vi "XLP80_Datalog_CreateFilename.vi"(8 "error in":errorcluster) -> (0 "error out":errorcluster caption="error in", 3 "Path":path, 5 "LogStartTime":dbl)   [LabVIEW 2021]
uses:
  XLP80_General_Libs/WL_Libs_V14.25/WL_Datalog_V14.00.llb/WL_Datalog_Global.vi
  XLP80_Globals/Globals_Settings_XLP80.vi
panel:
  out "x+1":i32
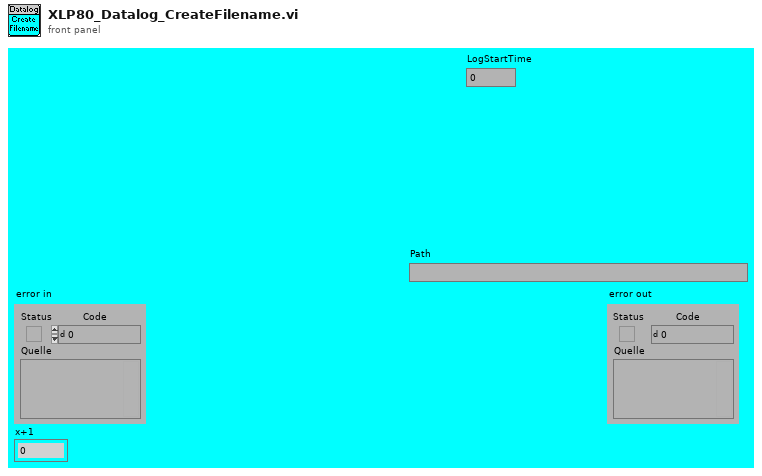
[diagram p1: front panel]
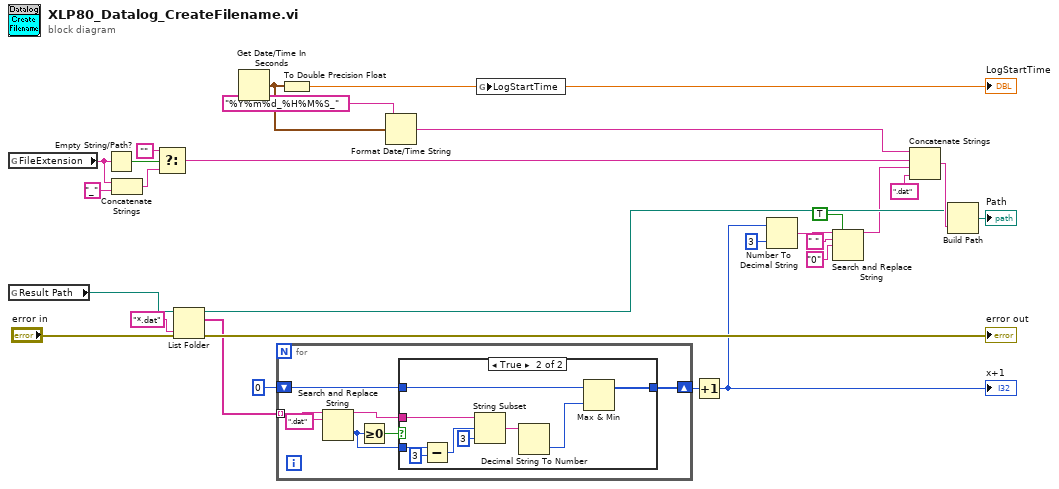
[diagram p0: block diagram]
diagram:
  n1 = global read "WL_Datalog_Global.vi" "FileExtension"() -> (w10:string)
  n2 = global read "Globals_Settings_XLP80.vi" "Result Path"() -> (w3:path)
  n3 = Empty String/Path?(string/path=w10) -> (empty?=w25:bool)
  n4 = Concatenate Strings(w10, "_" ("string")) -> (w24:string)
  n5 = Select(t="", s=w25, f=w24) -> (s? t:f=w1:string)
  n6 = List Folder(path=w3, pattern="*.dat", error in="error in") -> (path out=w13:path, filenames=w6:string[], error out=→"error out":errorcluster)  [unwired: 1 in, 1 out]
  n7 = Get Date/Time In Seconds() -> (seconds since 1Jan1904=w27:timestamp)
  n8 = for {
    tunnel: w6 -> [w35] mode=indexing
    shift-right: [w30] -> w5
    shift-left: 0 -> [w31]
    n9 = Search and Replace String(input string=w35, search string=".dat") -> (result string=w32:string, offset past replacement=w29:i32)  [unwired: 6 in, 2 out]
    n10 = Greater Or Equal To 0?(x=w29) -> (x >= 0?=w33:bool)
    n11 = case shown="True" w33 {
      tunnel: w32 -> [_ w43]
      tunnel: w31 -> [w36 w39]
      tunnel: [w36 w37] -> w30
      tunnel: w29 -> [_ w45]
      frame False {
      }
      frame True {
        n12 = Subtract(x=w45, y=3) -> (x-y=w42:i32)
        n13 = String Subset(string=w43, offset (0)=w42, length (rest)=3 ("length (rest)")) -> (substring=w40:string)
        n14 = Decimal String To Number(string=w40) -> (number=w38:i32)  [unwired: 2 in, 1 out]
        n15 = Max & Min(x=w39, y=w38) -> (max(x,y)=w37:i32)  [unwired: 1 out]
      }
    }
  }
  n16 = To Double Precision Float(number=w27) -> (double precision float=w20:dbl)
  "LogStartTime" <- w20
  n17 = Format Date/Time String(time format string (%c)="%Y%m%d_%H%M%S_", seconds (now)=w27) -> (date/time string=w2:string)  [unwired: 1 in]
  n18 = global write "WL_Datalog_Global.vi" "LogStartTime"(w20) -> ()
  n19 = Increment(x=w5) -> (x+1=w4:i32)
  "x+1" <- w4
  n20 = Number To Decimal String(number=w4, width (-)=i16 3) -> (decimal integer string=w16:string)
  n21 = Search and Replace String(replace all?=TRUE ("replace all? (F)"), input string=w16, search string=" ", replace string="0" ("replace string (\"\")")) -> (result string=w11:string)  [unwired: 4 in, 3 out]
  n22 = Concatenate Strings(w2, w1, w11, ".dat" ("string")) -> (w22:string)
  n23 = Build Path(base path=w13, name or relative path=w22) -> (appended path=→"Path":path)
